vi "Punto 2 _ JUAN BERMUDEZ.vi"() -> ()   [LabVIEW 2020]
panel:
  in  "stop":bool
  out "Vocales segunda mitad":i32
  out "Vocales primera mitad":i32
  out "Vocales totales, para resultado correcto, recuerde refrescar":i32
  in  "Accionar":bool
  out "Segunda mitad":string
  out "Primera mitad":string
  in  "Textro inicial":string
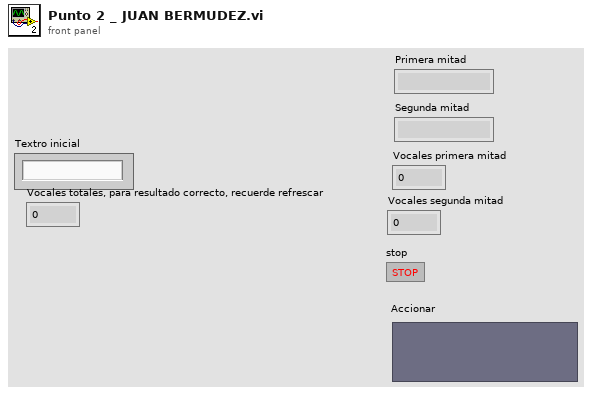
[diagram p1: front panel]
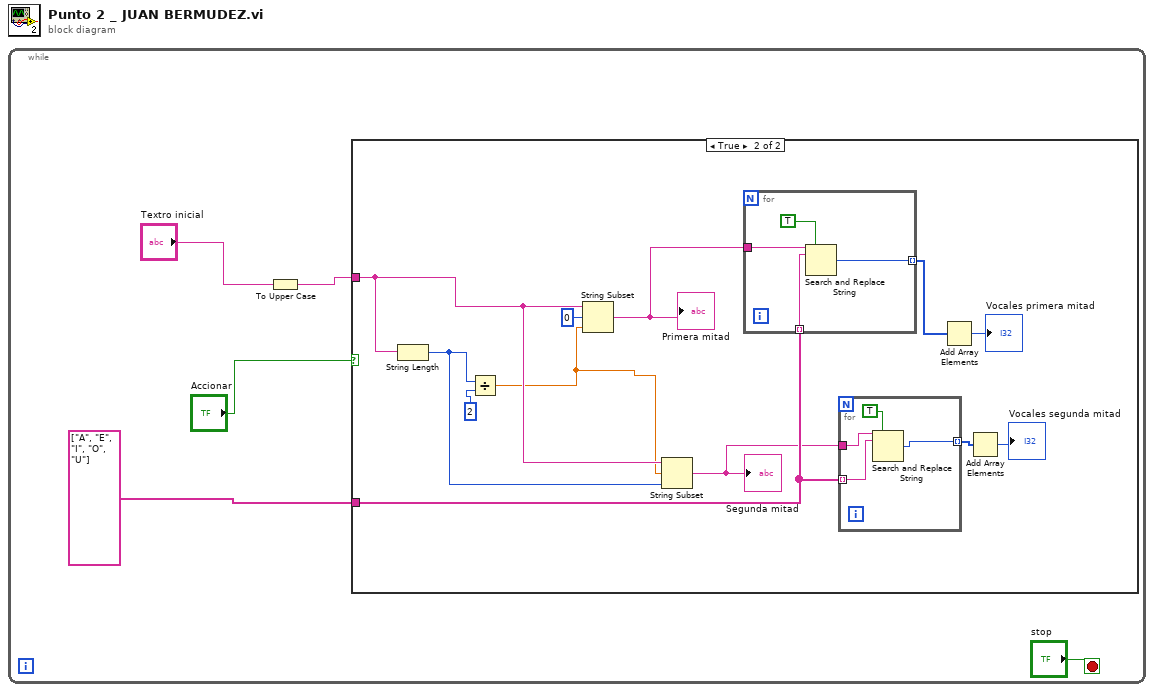
[diagram p0: block diagram]
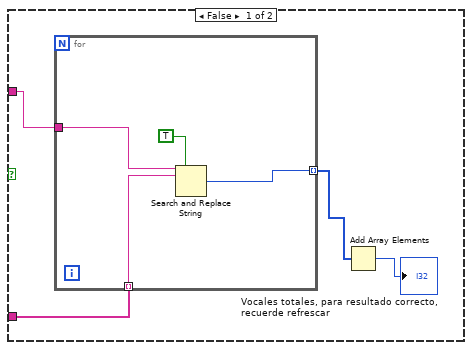
[diagram p2: hidden frame]
diagram:
  n1 = while {
    stop <- "stop" stop-if-true
    n2 = To Upper Case(1:"Textro inicial") -> (0:w5:string)
    n3 = case shown="True" "Accionar" {
      tunnel: w5 -> [w9 w23]
      tunnel: string[] ["A", "E", "I", "O", "U"] -> [w8 w19]
      frame False {
        n4 = for {
          tunnel: w9 -> [w10]
          tunnel: w8 -> [w13] mode=indexing
          tunnel: [w11] -> w7 mode=indexing
          n5 = Search and Replace String(replace all?=TRUE ("replace all? (F)"), input string=w10, search string=w13) -> (number of replacements=w11:i32)  [unwired: 5 in, 3 out]
        }
        n6 = Add Array Elements(numeric array=w7) -> (sum=→"Vocales totales, para resultado correcto, recuerde refrescar":i32)
      }
      frame True {
        n7 = String Length(string=w23) -> (length=w22:i32)
        n8 = Divide(x=w22, y=2) -> (x/y=w16:dbl)
        n9 = String Subset(string=w23, offset (0)=0, length (rest)=w16) -> (substring=w15:string)
        "Primera mitad" <- w15
        n10 = String Subset(string=w23, offset (0)=w16, length (rest)=w22) -> (substring=w14:string)
        "Segunda mitad" <- w14
        n11 = for {
          tunnel: w19 -> [w33] mode=indexing
          tunnel: [w32] -> w21 mode=indexing
          tunnel: w15 -> [w31]
          n12 = Search and Replace String(replace all?=TRUE ("replace all? (F)"), input string=w31, search string=w33) -> (number of replacements=w32:i32)  [unwired: 5 in, 3 out]
        }
        n13 = for {
          tunnel: w19 -> [w29] mode=indexing
          tunnel: [w28] -> w17 mode=indexing
          tunnel: w14 -> [w27]
          n14 = Search and Replace String(replace all?=TRUE ("replace all? (F)"), input string=w27, search string=w29) -> (number of replacements=w28:i32)  [unwired: 5 in, 3 out]
        }
        n15 = Add Array Elements(numeric array=w21) -> (sum=→"Vocales primera mitad":i32)
        n16 = Add Array Elements(numeric array=w17) -> (sum=→"Vocales segunda mitad":i32)
      }
    }
  }
